vi "K2400_I_mea.vi"(2 "error in":errorcluster, 3 "Adress (24)":string) -> (0 "error out":errorcluster, 1 "I (A)":dbl)   [LabVIEW 2021]
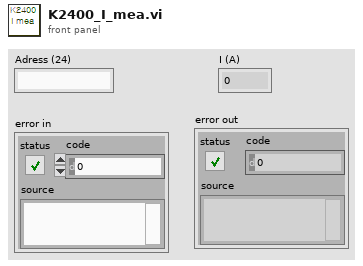
[diagram p1: front panel]
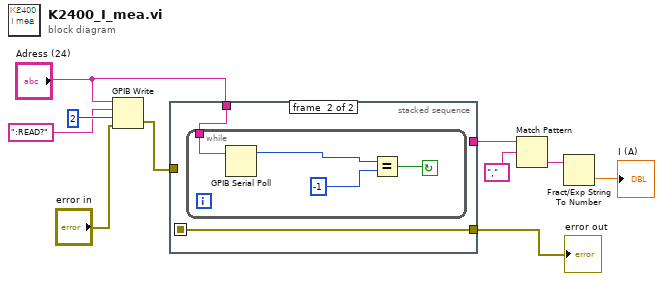
[diagram p0: block diagram]
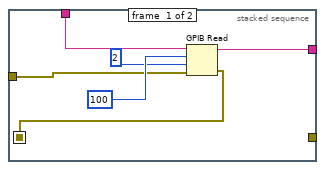
[diagram p2: hidden frame]
diagram:
  n1 = GPIB Write(0:"Adress (24)", 1:":READ?", 2:2, 3:"error in") -> (6:w8:errorcluster)  [unwired: 1 in, 1 out]
  n2 = stacked-sequence {
    seq-local: [w15 _] -> [_ w17]
    tunnel: w8 -> [w13 _]
    tunnel: "Adress (24)" -> [w11 w18]
    tunnel: [w12 _] -> w6
    tunnel: [_ w17] -> w1
    frame #0 {
      n3 = GPIB Read(0:w11, 1:100, 2:2, 3:w13) -> (5:w12:string, 7:w15:errorcluster)  [unwired: 1 in, 1 out]
    }
    frame #1 {
      n4 = while {
        tunnel: w18 -> [w21]
        stop <- w22 continue-if-true
        n5 = GPIB Serial Poll(0:w21) -> (2:w20:i16)  [unwired: 1 in, 2 out]
        n6 = Equal?(x=w20, y=-1) -> (x = y?=w22:bool)
      }
    }
  }
  "error out" <- w1
  n7 = Match Pattern(string=w6, regular expression=",") -> (after substring=w5:string)  [unwired: 1 in, 3 out]
  n8 = Fract/Exp String To Number(string=w5) -> (number=→"I (A)":dbl)  [unwired: 3 in, 1 out]
